vi "SavedSettingsSetAllIcons.vi"(11 "TreeControl in":refnum<vi>) -> ()   [LabVIEW 2021]
panel:
  out "error out":errorcluster
  in  "error in (no error)":errorcluster
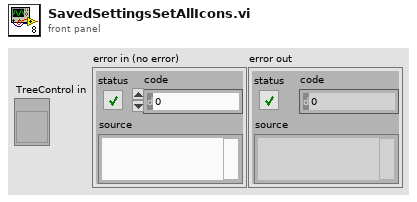
[diagram p1: front panel]
types:
  T1 = typedef "SavedSettingsOptions.ctl" = cluster{"OpenVIs":bool, "RunVIs":bool, "RestoreSubItems":bool, "WaitAfter":u32}
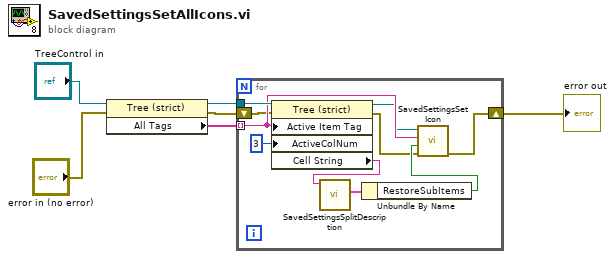
[diagram p0: block diagram]
diagram:
  n1 = property class="Tree (strict)"(reference="TreeControl in", error in="error in (no error)") -> (reference out=w4:refnum<vi>, error out=w6:errorcluster, "All Tags"=w5:string[])
  n2 = for {
    tunnel: w4 -> [w15]
    tunnel: w5 -> [w11] mode=indexing
    shift-right: [w7] -> w1
    shift-left: w6 -> [w8]
    n3 = property class="Tree (strict)"(reference=w15, error in=w8, "Active Item Tag"=w11, "ActiveColNum"=3 ("Active Cell:Active Column Number")) -> (reference out=w10:refnum<vi>, error out=w9:errorcluster, "Cell String"=w13:string)
    n4 = call "SavedSettingsSplitDescription.vi"("Description in"=w13) -> ("Options"=w16:T1)  [unwired: 9 in, 1 out]
    n5 = Unbundle By Name(w16) -> ("RestoreSubItems"=w12:bool)
    n6 = call "SavedSettingsSetIcon.vi"("error in (no error)"=w9, "Restore SubItems"=w12, "Tag"=w11, "TreeControl in"=w10) -> ("error out"=w7:errorcluster)  [unwired: 6 in, 1 out]
  }
  "error out" <- w1
